vi "CRY1DArray data.vi"(11 "Array":dbl[](array[numeric])) -> ()   [LabVIEW 2013]
panel:
  out "Numeric":i32
  out "XY Graph":cluster{i32[], "Array":dbl[]}(graph) caption="Stimulus_Ear_Graph"
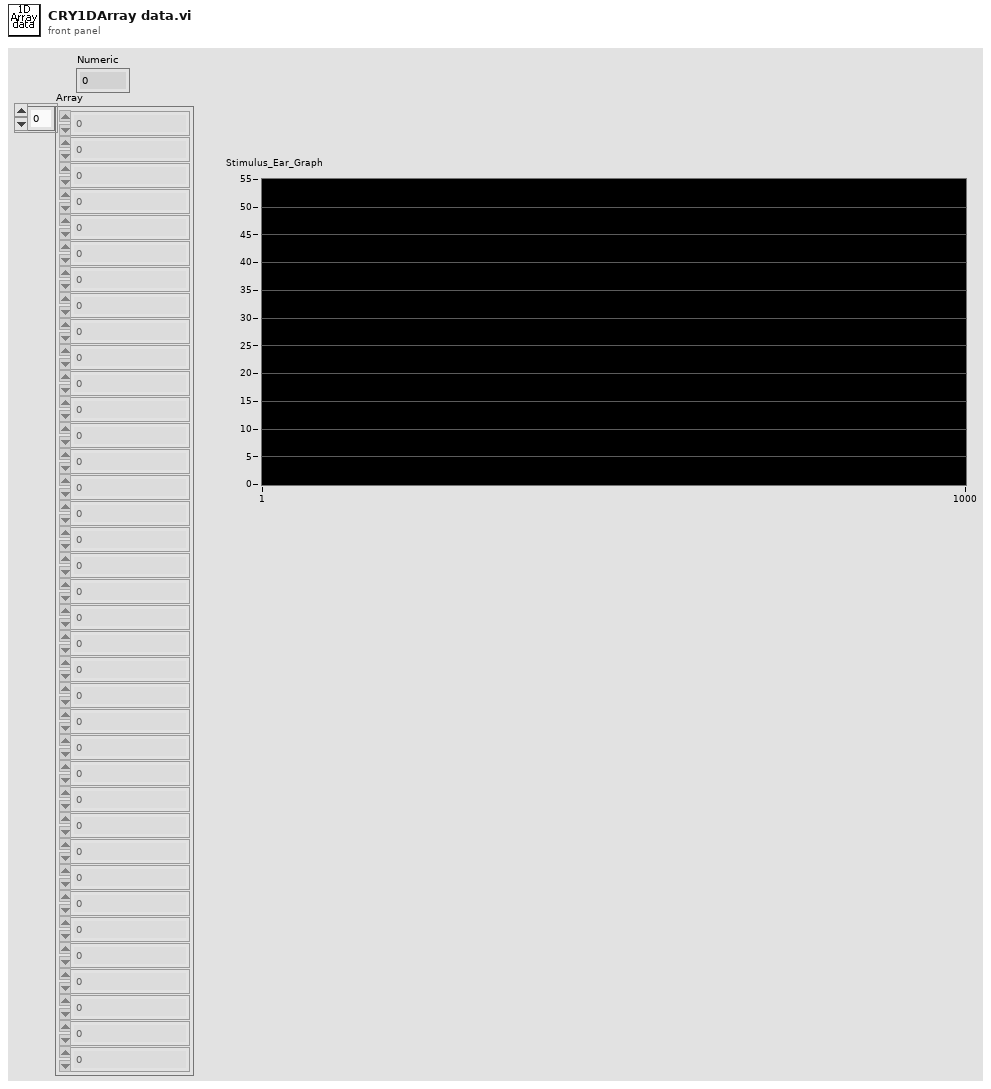
[diagram p1: front panel]
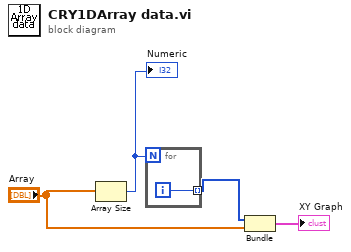
[diagram p0: block diagram]
diagram:
  n1 = Array Size(array="Array") -> (size(s)=w1:i32)
  "Numeric" <- w1
  n2 = for {
    N: w1 -> [_]
    tunnel: [w5] -> w3 mode=indexing
    i -> [w5]
  }
  n3 = Bundle(w3, "Array"="Array") -> (→"XY Graph":cluster{i32[], "Array":dbl[]})  [unwired: 1 out]
